vi "不合格信息录入.vi"(0 "不合格代码":string, 1 "功能":enum16{"录入", "清空"}(ring), 11 "错误输入（无错误）":errorcluster) -> (15 "错误输出":errorcluster)   [LabVIEW 2020]
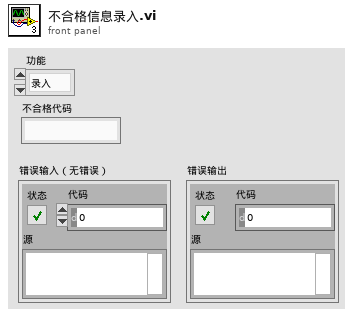
[diagram p1: front panel]
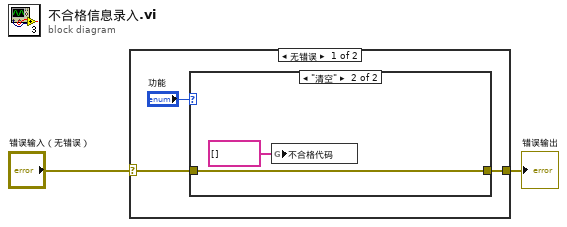
[diagram p0: block diagram]
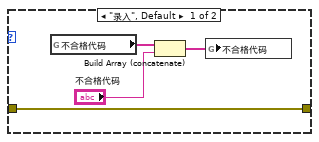
[diagram p2: hidden frame]
diagram:
  n1 = case shown="无错误" "错误输入（无错误）" {
    selector: "错误输入（无错误）" -> [w4 w12]
    tunnel: [w3 w12] -> w1
    frame No Error {
      n2 = case shown="\"清空\"" "功能" {
        tunnel: [w8 w10] -> w3
        tunnel: w4 -> [w8 w10]
        frame "录入", Default {
          n3 = global read "追溯全部变量.vi" "不合格代码"() -> (w7:string[])
          n4 = Build Array (concatenate)(w7, "不合格代码") -> (w6:string[])
          n5 = global write "追溯全部变量.vi" "不合格代码"(w6) -> ()
        }
        frame "清空" {
          n6 = global write "追溯全部变量.vi" "不合格代码"(string[] [] ("不合格代码")) -> ()
        }
      }
    }
    frame Error {
    }
  }
  "错误输出" <- w1
